vi "Set rolling shutter pace.vi"(8 "error in (no error)":errorcluster, 11 "DAQOrcaFlash in":refnum<class "DAQOrcaFlash.lvclass">) -> (0 "error out":errorcluster, 3 "DAQOrcaFlash out":refnum<class "DAQOrcaFlash.lvclass">)   [LabVIEW 2012, in "DAQOrcaFlash.lvclass"]
uses:
  DAQOrcaFlash.lvclass
  DAQOrcaFlash.lvclass/DAQOrcaFlash.ctl
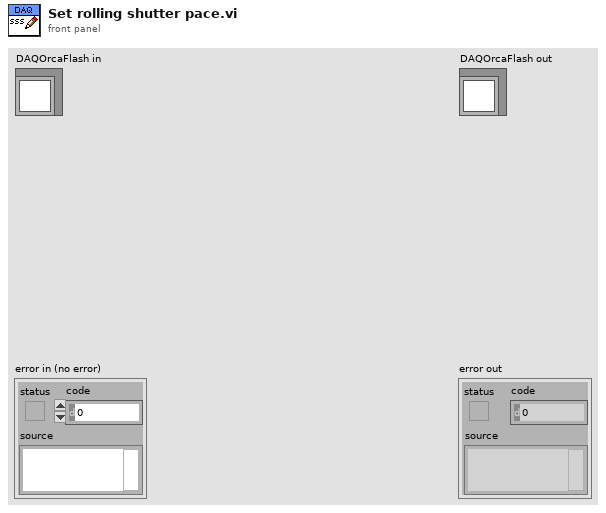
[diagram p1: front panel]
types:
  T1 = typedef "DAQOrcaFlash.lvclass/sensor_mode.ctl" = sgl
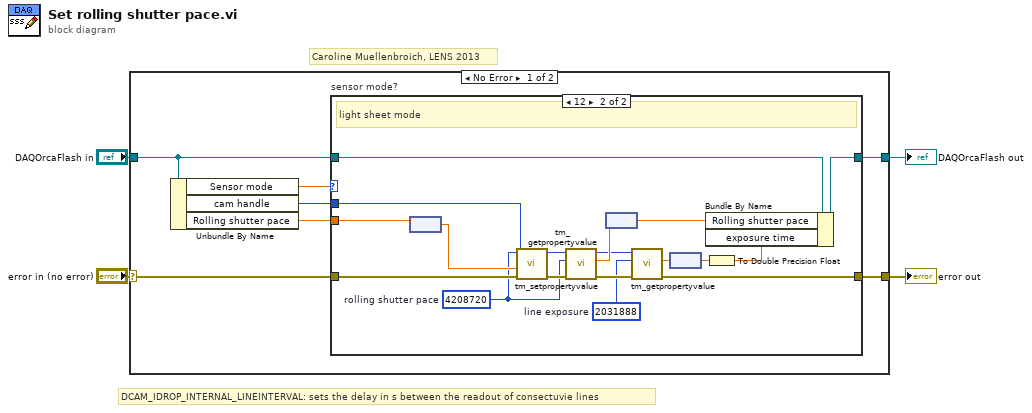
[diagram p0: block diagram]
diagram:
  # "DCAM_IDROP_INTERNAL_LINEINTERVAL: sets the delay in s between the readout of consectuvie lines"
  # "Caroline Muellenbroich, LENS 2013"
  n1 = case shown="No Error" "error in (no error)" {
    selector: "error in (no error)" -> [w11 w33]
    tunnel: [w7 w33] -> w3
    tunnel: [w5 w32] -> w1
    tunnel: "DAQOrcaFlash in" -> [w6 w32]
    frame No Error {
      n2 = Unbundle By Name(w6) -> ("Sensor mode"=w8:T1, "cam handle"=w10:u32, "Rolling shutter pace"=w9:sgl[unit])
      n3 = case "sensor mode?" shown="12" w8 {
        tunnel: [w13 w21] -> w7
        tunnel: w11 -> [w13 w31]
        tunnel: w10 -> [_ w30]
        tunnel: w9 -> [_ w29]
        tunnel: w6 -> [w12 w16]
        tunnel: [w12 w14] -> w5
        frame 1, Default {
          # "frame imaging"
        }
        frame 12 {
          w20 = u32 2031888  # line exposure
          w25 = u32 4208720  # rolling shutter pace
          # "light sheet mode"
          n4 = node(w29) -> (w28:sgl)
          n5 = call <userlib>:"tm_setpropertyvalue.vi"("error in (no error)"=w31, "Value in"=w28, "Property ID"=w25, "Handle in"=w30) -> ("error out"=w27:errorcluster, "Handle out"=w26:u32)  [unwired: 6 in]
          n6 = call <userlib>:"tm_getpropertyvalue.vi"("error in (no error)"=w27, "Property ID"=w25, "Handle in"=w26) -> ("error out"=w22:errorcluster, "Value in"=w24:sgl, "Handle out"=w23:u32)  [unwired: 6 in]
          n7 = node(w24) -> (w18:sgl[unit])
          n8 = call <userlib>:"tm_getpropertyvalue.vi"("error in (no error)"=w22, "Property ID"=w20, "Handle in"=w23) -> ("error out"=w21:errorcluster, "Value in"=w19:sgl)  [unwired: 6 in, 1 out]
          n9 = node(w19) -> (w17:sgl[unit])
          n10 = To Double Precision Float(number=w17) -> (double precision float=w15:dbl[unit])
          n11 = Bundle By Name(cluster=w16, "Rolling shutter pace"=w18, "exposure time"=w15) -> (w14:refnum<class "DAQOrcaFlash.lvclass">)
        }
      }
    }
    frame Error {
    }
  }
  "error out" <- w3
  "DAQOrcaFlash out" <- w1
